vi "Calibration.vi"(0 "Mode":T3, 5 "Calib file":path, 9 "Simulate/Run":T2) -> (14 "Calib const":string[][](array[string]), 16 "Coefficients":dbl[][](array[numeric]) format="%.2f", 19 "Status Out":T1)   [LabVIEW 2015]
uses:
  Anemometry Sub Vis/Globals/Calib_global.vi
  Anemometry Sub Vis/Globals/Meas_global.vi
  Anemometry Sub Vis/Controls/Setup.ctl
  Anemometry Sub Vis/Controls/Post_Process.ctl
  Anemometry Sub Vis/Gen Trav/Multi_Run_Status.ctl
  Anemometry Sub Vis/Controls/App_Global.ctl
  Anemometry Sub Vis/Calibration/Calib_mode.ctl
  Anemometry Sub Vis/Controls/Save_Data.ctl
  Anemometry Sub Vis/Acquisition/PWA/PWAtasksGLOBAL.vi
  Anemometry Sub Vis/File/Setup_Filetype.ctl
  <vilib>/Analysis/NI_AALBase.lvlib
  <vilib>/Analysis/baseanly.llb/Mean (DBL).vi
  Anemometry Sub Vis/Controls/User_Specific_mode.ctl
panel:
  in  "-ve Ref Values":bool
  out "String":string
  in  "polynomial order":i32=2 min=1 max=3 step=1
  out "Ref velocity":dbl[](array[numeric])=[2.4275346736, 2.4395664609, 2.453235235, 2.4247395837, 2.4277603784, 2.41169823, 2.4254144559, 2.424896502176921] format="%.3f"
  out "labels":string[](array[string])=["XW1 Volt", "XW2 Volt", "Entered Val", "Selector"]
  in  "Point selector 3":cluster{"Y":dbl, "X":dbl, "t/f":bool}[](array[cluster]) {"X" format="%#.2g"; "Y" format="%#.3f"}
  in  "n":dbl=0.45 format="%.4f"
  in  "Fixed n":bool=TRUE
  out "Sample of input signals":dbl[][](graph)
  in  "Sampling speeds":T4={"Samples/ch"=600, "Sample Rate/ch (Hz)"=100.0} {"Sample Rate/ch (Hz)" min=0; "Samples/ch" min=0 step=1}
  out "Calibration plot":cluster{cluster{dbl, dbl}[]}[](graph)
  in  "Point selector 4":T5(array[cluster]) {"Y2" format="%#.2f"; "X" format="%#.3f"; "Y" format="%#.2f"}
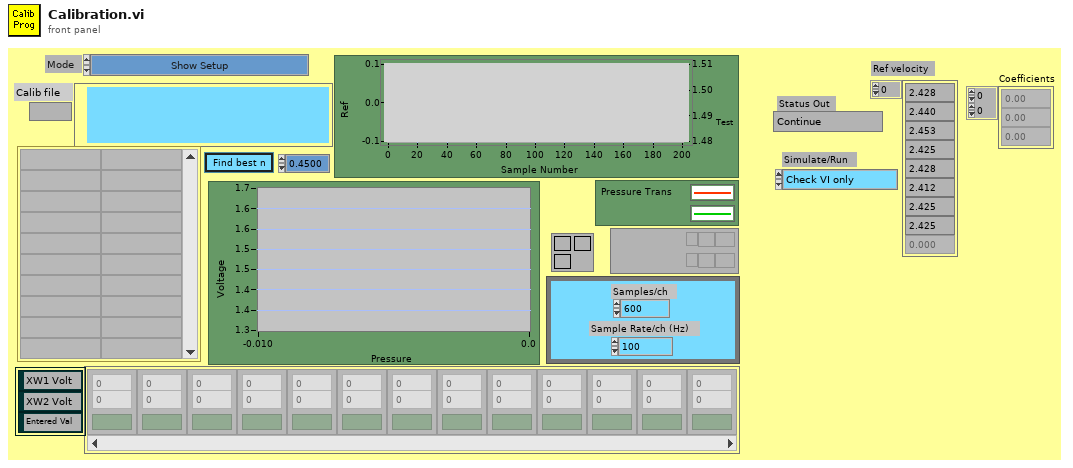
[diagram p1: front panel]
types:
  T1 = typedef "Multi_Run_Status.ctl" = enum16{"Continue", "Jump to Next Point", "Jump to Next Row", "Jump To Fall Back", "Terminate Run"}
  T2 = typedef "User_Specific_mode.ctl" = enum16{"Check VI only", "Run VI"}
  T3 = typedef "Calib_mode.ctl" = enum16{"Show Setup", "Take a New Calibration Point", "Refit Curve", "Setup Front Panel"}
  T4 = cluster{"Samples/ch":i32, "Sample Rate/ch (Hz)":sgl}
  T5 = cluster{"Y":dbl, "Y2":dbl, "X":dbl, "t/f":bool}[]
  T6 = typedef "Post_Process.ctl" = enum16{"Take New Data", "Post Process Raw Data File"}
  T7 = typedef "Setup_Filetype.ctl" = enum16{"Measurement Setups", "Calibration Setups", "General", "Results File Plotter Setups", "Speed Calib Tweaks"}
  T8 = typedef "Save_Data.ctl" = enum16{"Save No Data", "Save Data"}
  T9 = typedef "Setup.ctl" = enum16{"Run Program", "Show Setup", "Save Current Setup", "Setup Front Panel"}
  T10 = typedef "App_Global.ctl" = enum16{"Read Global", "Write to Global", "Initialise Array"}
  T11 = enum32{"existing file", "new file", "new or existing file", "existing dir", "new dir", "new or existing dir", "existing file (use LLBs)", "new file (use LLBs)", "new or existing file (use LLBs)", "new or existing file or directory (use LLBs)"}
  T12 = cluster{"Samples /ch":i32, "Sampling Rate /ch (Hz)":sgl}
  T13 = typedef "Cal_Inst_type.ctl" = enum16{"Propeller anemometer", "Pressure Transducer", "Hot wire", "Cross wire velocity", "Cross wire angle", "Generic Linear", "Generic Polynomial", "Generic BackPoly", "Fast FID", "Thermocouple", "Cold wire", "Pulsed Wire"}
  T14 = typedef "Ref_Inst_type.ctl" = enum16{"Propellor anemometer", "Pressure Transducer", "Raw voltage", "Pitot-static tube", "Preston tube", "Generic Linear", "Generic Polynomial", "Thermocouple", "LDA", "Enter Value", "ADAM Channel"}
  T15 = cluster{"2nd Ref type":T14, "2nd inst present":bool}
  T16 = typedef "Analysis_info_cluster.ctl" = cluster{"Colour":u32, "Inst type":T17, "Inst name":string, "Symbol":string, "Code name":string, "Extra Info":string, "Inst Array":T18, "Extra Titles":string[], "Extra Values":string[], "U":dbl, "u^2":dbl, "u^3":dbl, "u^4":dbl, "Skew_u":dbl, "Kurt_u":dbl, "Sd Error in Mean":dbl, "% u'/U":dbl, "X":dbl, "Y":dbl, "Z":dbl, "Timescale integral to 25%":dbl, "Sd Error in Variance":dbl, "Calib File":path, "Calib Constants":dbl[], "Output Position":bool, "Full Stats":bool, "Av Sampling Rate":dbl, "Av No of Samples":dbl, "Total Meas Time (s)":dbl, "ADAM Ch Name":string}
  T17 = typedef "Inst_type.ctl" = enum16{"Propeller anemometer", "Raw voltage", "Pressure Transducer", "Pitot-static tube", "Preston tube", "Hot wire", "Cross wire 1", "Cross wire 2", "Generic Linear", "Generic Polynomial", "Generic BackPoly", "Fast FID", "Thermocouple", "Cold wire", "Pulsed Wire", "LDA Vel", "LDA Tran time", "LDA Arr time", "Microphone"}
  T18 = typedef "Instrument_Array.ctl" = enum16{"PWA", "LDA", "Analogue"}
  T19 = typedef "Time_Trace_Cluster.ctl" = cluster{"Weighting":dbl[], "Time (s)":dbl[], "Voltage":dbl[], "Eng Values":dbl[]}
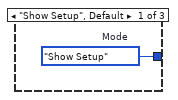
[diagram p5: hidden frame]
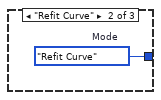
[diagram p6: hidden frame]
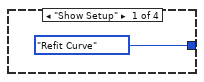
[diagram p7: hidden frame]
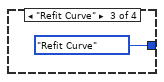
[diagram p8: hidden frame]
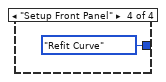
[diagram p9: hidden frame]
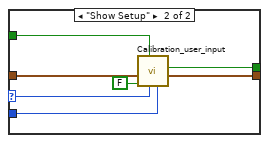
[diagram p14: hidden frame]
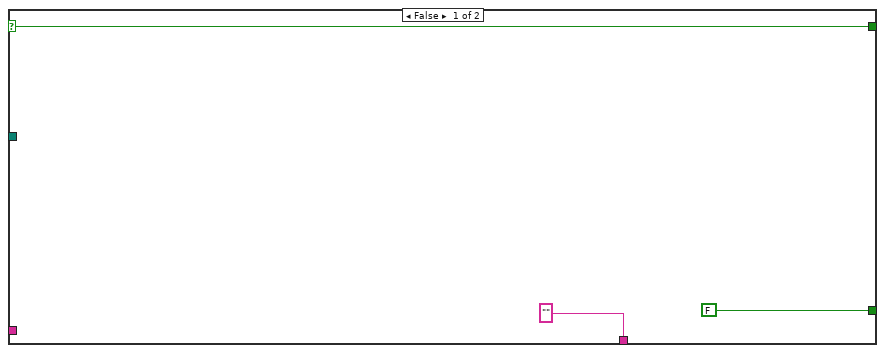
[diagram p15: hidden frame]
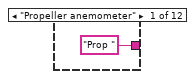
[diagram p16: hidden frame]
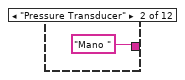
[diagram p17: hidden frame]
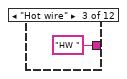
[diagram p18: hidden frame]
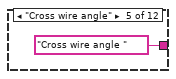
[diagram p19: hidden frame]
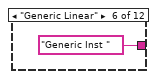
[diagram p20: hidden frame]
diagram:
  # "Change of file"
  # "Take new point"
  # "Calib File already valid"
  # "Main Calib File"
  # "Temp"
  # "Temp"
  # "Setup"
  # "E inst 1"
  # "Ref"
  # "E Inst 1\n+ 1 pt"
  # "Vel\n+1 pt"
  # "E inst 2"
  # "E Inst 2\n+ 1 pt"
  # "2nd ref"
  # "2nd ref"
  n1 = flat-sequence {
    tunnel: "Simulate/Run" -> [w106]
    tunnel: [w115] -> w101
    tunnel: [w120] -> w100
    tunnel: [w114] -> w99
    tunnel: w101 -> [w134]
    tunnel: [w134] -> w98
    tunnel: w100 -> [w129]
    tunnel: [w129] -> w97
    tunnel: [w136] -> w96
    tunnel: [w130] -> w95
    tunnel: [w133] -> w94
    tunnel: w99 -> [w128]
    tunnel: [w128] -> w93
    tunnel: w98 -> [w153]
    tunnel: [w153] -> w92
    tunnel: w97 -> [w152]
    tunnel: [w152] -> w91
    tunnel: w96 -> [w157]
    tunnel: [w157] -> w90
    tunnel: w95 -> [w156]
    tunnel: [w156] -> w89
    tunnel: w94 -> [w154]
    tunnel: [w154] -> w88
    tunnel: w93 -> [w151]
    tunnel: [w151] -> w87
    tunnel: [w189] -> w86
    tunnel: [w190] -> w85
    tunnel: w92 -> [w188]
    tunnel: [w188] -> w84
    tunnel: w91 -> [w187]
    tunnel: [w182] -> w83
    tunnel: w90 -> [w185]
    tunnel: [w185] -> w82
    tunnel: w89 -> [w184]
    tunnel: [w184] -> w81
    tunnel: w88 -> [w183]
    tunnel: [w183] -> w80
    tunnel: w87 -> [w186]
    tunnel: [w186] -> w79
    tunnel: w86 -> [w240]
    tunnel: [w240] -> w78
    tunnel: w85 -> [w239]
    tunnel: [w239] -> w77
    tunnel: w84 -> [w238]
    tunnel: [w238] -> w76
    tunnel: w83 -> [w237]
    tunnel: [w237] -> w75
    tunnel: w82 -> [w236]
    tunnel: [w236] -> w74
    tunnel: w81 -> [w235]
    tunnel: [w235] -> w73
    tunnel: w80 -> [w234]
    tunnel: [w234] -> w72
    tunnel: w79 -> [w233]
    tunnel: [w233] -> w71
    tunnel: w78 -> [w371]
    tunnel: [w371] -> w70
    tunnel: w77 -> [w370]
    tunnel: [w370] -> w69
    tunnel: w76 -> [w369]
    tunnel: [w369] -> w68
    tunnel: w75 -> [w368]
    tunnel: [w368] -> w67
    tunnel: w74 -> [w367]
    tunnel: [w367] -> w66
    tunnel: w73 -> [w366]
    tunnel: [w366] -> w65
    tunnel: w72 -> [w365]
    tunnel: [w365] -> w64
    tunnel: w71 -> [w364]
    tunnel: [w364] -> w63
    tunnel: [w510] -> w62
    tunnel: [w509] -> w61
    tunnel: [w508] -> w60
    tunnel: [w507] -> w59
    tunnel: w70 -> [w496]
    tunnel: w69 -> [w497]
    tunnel: [w506] -> w58
    tunnel: w68 -> [w490]
    tunnel: [w490] -> w57
    tunnel: w67 -> [w489]
    tunnel: [w489] -> w56
    tunnel: w66 -> [w488]
    tunnel: [w488] -> w55
    tunnel: w65 -> [w487]
    tunnel: [w487] -> w54
    tunnel: [w498] -> w53
    tunnel: w64 -> [w486]
    tunnel: [w486] -> w52
    tunnel: w63 -> [w491]
    tunnel: w62 -> [w543]
    tunnel: [w543] -> w51
    tunnel: w61 -> [w542]
    tunnel: [w542] -> w50
    tunnel: w60 -> [w541]
    tunnel: [w541] -> w49
    tunnel: w59 -> [w540]
    tunnel: [w540] -> w48
    tunnel: w58 -> [w539]
    tunnel: [w539] -> w47
    tunnel: w57 -> [w538]
    tunnel: [w538] -> w46
    tunnel: w56 -> [w547]
    tunnel: w55 -> [w537]
    tunnel: [w537] -> w45
    tunnel: w54 -> [w536]
    tunnel: [w536] -> w44
    tunnel: w53 -> [w545]
    tunnel: w52 -> [w544]
    tunnel: w51 -> [w569]
    tunnel: [w569] -> w43
    tunnel: w50 -> [w568]
    tunnel: [w568] -> w42
    tunnel: w49 -> [w567]
    tunnel: [w567] -> w41
    tunnel: w48 -> [w566]
    tunnel: [w566] -> w40
    tunnel: w47 -> [w565]
    tunnel: [w565] -> w39
    tunnel: w46 -> [w564]
    tunnel: [w564] -> w38
    tunnel: w45 -> [w563]
    tunnel: [w563] -> w37
    tunnel: w44 -> [w571]
    tunnel: [w571] -> w36
    tunnel: w43 -> [w616]
    tunnel: [w616] -> w35
    tunnel: w42 -> [w615]
    tunnel: [w615] -> w34
    tunnel: w41 -> [w614]
    tunnel: [w614] -> w33
    tunnel: w40 -> [w613]
    tunnel: [w613] -> w32
    tunnel: [w620] -> w31
    tunnel: w39 -> [w612]
    tunnel: [w612] -> w30
    tunnel: w38 -> [w621]
    tunnel: [w621] -> w29
    tunnel: w37 -> [w611]
    tunnel: [w611] -> w28
    tunnel: w36 -> [w610]
    tunnel: [w610] -> w27
    tunnel: [w647] -> w26
    tunnel: [w646] -> w25
    tunnel: w35 -> [w649]
    tunnel: w34 -> [w648]
    tunnel: w33 -> [w644]
    tunnel: [w645] -> w24
    tunnel: w32 -> [w643]
    tunnel: [w642] -> w23
    tunnel: w31 -> [w635]
    tunnel: [w635] -> w22
    tunnel: [w640] -> w21
    tunnel: w30 -> [w633]
    tunnel: w29 -> [w638]
    tunnel: [w638] -> w20
    tunnel: w28 -> [w637]
    tunnel: [w637] -> w19
    tunnel: w27 -> [w634]
    tunnel: [w634] -> w18
    tunnel: w26 -> [w995]
    tunnel: w25 -> [w998]
    tunnel: [w998] -> w17
    tunnel: w24 -> [w997]
    tunnel: w23 -> [w992]
    tunnel: w22 -> [w990]
    tunnel: [w990] -> w16
    tunnel: w21 -> [w996]
    tunnel: w20 -> [w989]
    tunnel: [w989] -> w15
    tunnel: w19 -> [w988]
    tunnel: [w988] -> w14
    tunnel: w18 -> [w987]
    tunnel: [w987] -> w13
    tunnel: [w993] -> w12
    tunnel: [w991] -> w11
    tunnel: w17 -> [w1009]
    tunnel: [w1009] -> w10
    tunnel: w16 -> [w1008]
    tunnel: [w1008] -> w9
    tunnel: w15 -> [w1026]
    tunnel: [w1026] -> w8
    tunnel: w14 -> [w1007]
    tunnel: [w1007] -> w7
    tunnel: w13 -> [w1006]
    tunnel: [w1006] -> w6
    tunnel: w12 -> [w1010]
    tunnel: w11 -> [w1025]
    tunnel: w10 -> [w1042]
    tunnel: [w1042] -> w5
    tunnel: w9 -> [w1047]
    tunnel: w8 -> [w1039]
    tunnel: [w1039] -> w4
    tunnel: w7 -> [w1041]
    tunnel: [w1041] -> w3
    tunnel: w6 -> [w1040]
    tunnel: [w1040] -> w2
    tunnel: w5 -> [w1069]
    tunnel: w4 -> [w1070]
    tunnel: w3 -> [w1071]
    tunnel: w2 -> [w1068]
    tunnel: [w1068] -> w1
    tunnel: w1 -> [w1117]
    frame #0 {
      w104 = FALSE  # Visible
      # "Calib-Frame0-InitialSetup"
      n2 = case shown="\"Run VI\"" w106 {
        frame "Check VI only" {
        }
        frame "Run VI" {
          n3 = Current VI's Path() -> (path=w108:path)
          n4 = call "Open_Close_Front_Panel.ph.vi"("Front Panel Window:Open"=TRUE, "VI path"=w108) -> ()  [unwired: 2 out]
        }
      }
      n5 = call "Run_EnFlo_Hub.vi"() -> ()  [unwired: 8 out]
      n6 = property on="String" class="Str"("Visible"=w104, "Blinking"=w104) -> ()  [unwired: 2 in, 2 out]
      n7 = global write "Calib_global.vi" "New Setup String"("") -> ()
      n8 = global write "Meas_global.vi" "Raw data option"(enum16{"Save raw data", "Raw data not saved"}."Save raw data" ("Raw data option")) -> ()
      n9 = global write "Meas_global.vi" "Post Process"(Post_Process."Take New Data" ("Post Process")) -> ()
    }
    frame #1 {
      w121 = FALSE  # Warn if Already Exists
      # "Calib-Frame1-FrameDescription"
      n10 = call "Current_Filepath.vi"("Short_Name"="Cal" ("Data Type"), "Filename in"="Calib file", "Data Type"="Calibrations") -> ("Filename Out"=w112:path)  [unwired: 1 in, 1 out]
      n11 = Empty String/Path?(string/path=w112) -> (empty?=w117:bool)
      n12 = case shown="True" w117 {
        tunnel: w112 -> [w123 _]
        tunnel: [w123 w125] -> w119
        frame False {
        }
        frame True {
          (unwired) T11."new or existing file" ("select mode (2)")
          # "Why is this here?"
          n13 = File Dialog(7:"Please Choose a new or existing Calibration filename" ("Promp if not found")) -> (1:w124:bool, 3:w125:path)  [unwired: 1 in, 7 out]
          n14 = Stop(stop? (T)=w124) -> ()
        }
      }
      n15 = call "Results_filename_checker.vi"("Warn if Already Exists"=w121, "Comment"="for the Calibration Prog", "Results file"=w119) -> ("exists?"=w120:bool, "cancelled"=w118:bool, "Results file output"=w115:path)  [unwired: 2 in, 1 out]
      n16 = Stop(stop? (T)=w118) -> ()
      n17 = global write "Calib_global.vi" "Calib file"(w115) -> ()
      n18 = local write "Calib file"(w115) -> ()
      n19 = global write "Meas_global.vi" "Results file"(w115) -> ()
      n20 = Format Into String(format string="Calibration File   %s", w115) -> (resulting string=w114:string)  [unwired: 2 in, 1 out]
    }
    frame #2 {
      # "Calib-Frame2-FrameDescription"
      n21 = while {
        shift-right: [w145] -> _
        shift-left: _ -> [w146]
        tunnel: w134 -> [w145]
        tunnel: [w144] -> w133
        stop <- FALSE continue-if-true
        n22 = Not Equal?(x=w146, y=w145) -> (x != y?=w144:bool)
      }
      n23 = Current VI's Path() -> (path=w135:path)
      n24 = call "Running_as_top_level.vi"("Vi path name"=w135) -> ("Top Level"=w127:bool)  [unwired: 1 out]
      n25 = Compound Arithmetic op=AND(w133, w127) -> (w132:bool)
      n26 = case shown="True" w132 {
        tunnel: "Mode" -> [w137 w138]
        tunnel: [w137 w139] -> w130
        frame False {
        }
        frame True {
          n27 = case shown="\"Setup Front Panel\"" w138 {
            selector: w138 -> [_ _ w142]
            tunnel: [w140 w141 w142] -> w139
            frame "Show Setup", Default {
              w140 = Calib_mode."Show Setup"  # Mode
            }
            frame "Refit Curve" {
              w141 = Calib_mode."Refit Curve"  # Mode
            }
            frame "Setup Front Panel" {
            }
          }
        }
      }
      n28 = case shown="\"Take a New Calibration Point\"" w130 {
        tunnel: [enum16{"Take new data point", "Refit Curve"}."Refit Curve" ("data mode") enum16{"Take new data point", "Refit Curve"}."Take new data point" ("data mode") enum16{"Take new data point", "Refit Curve"}."Refit Curve" ("data mode") enum16{"Take new data point", "Refit Curve"}."Refit Curve" ("data mode")] -> w136
        frame "Show Setup" {
        }
        frame "Take a New Calibration Point" {
        }
        frame "Refit Curve" {
        }
        frame "Setup Front Panel" {
        }
      }
    }
    frame #3 {
      # "The code in these two cases is essentially duplicated. Only,\nthe input to the Boolean input named \"OK\" differs between\nthe two cases. We should be able either flatten this out, or\nuse the case structure to only alter the input to the \"OK\"\ninput of Calibration_user_input.vi."
      # "Calib-Frame3-FrameDescription"
      n29 = local read "Fixed n"() -> (w159:bool)
      n30 = case shown="\"Setup Front Panel\"" w156 {
        tunnel: [w162 w163 TRUE w165] -> w155
        tunnel: w154 -> [w162 w163 _ w165]
        frame "Show Setup" {
        }
        frame "Refit Curve" {
        }
        frame "Setup Front Panel" {
        }
        frame "Take a New Calibration Point" {
        }
      }
      n31 = case shown="\"Take a New Calibration Point\", Default" w156 {
        selector: w156 -> [w168 w175]
        tunnel: "Sampling speeds" -> [w174 w181]
        tunnel: w157 -> [w172 w179]
        tunnel: [w171 w178] -> w160
        tunnel: w159 -> [w169 w177]
        tunnel: [w170 w176] -> w158
        frame "Take a New Calibration Point", Default {
          n32 = call "Calibration_user_input.vi"("data mode"=w172, "Mode"=w168, "Fixed n"=w169, "OK"=TRUE, "Sampling speeds"=w174) -> ("Sampling speeds Output"=w171:T12, "Fixed n out"=w170:bool)  [unwired: 2 in, 3 out]
        }
        frame "Show Setup" {
          n33 = call "Calibration_user_input.vi"("data mode"=w179, "Mode"=w175, "Fixed n"=w177, "OK"=FALSE, "Sampling speeds"=w181) -> ("Sampling speeds Output"=w178:T12, "Fixed n out"=w176:bool)  [unwired: 5 out]
        }
      }
      n34 = case shown="True" w155 {
        tunnel: w160 -> [_ w167]
        tunnel: w158 -> [_ w166]
        frame False {
        }
        frame True {
          n35 = local write "Sampling speeds"(w167) -> ()
          n36 = local write "Fixed n"(w166) -> ()
        }
      }
    }
    frame #4 {
      # "Calib-Frame4-FrameDescription"
      n37 = case shown="True" w187 {
        selector: w187 -> [w191 w194]
        tunnel: ["" ("Output string") w209] -> w190
        tunnel: [FALSE w208] -> w189
        tunnel: w188 -> [_ w200]
        tunnel: w186 -> [_ w195]
        tunnel: [w191 w194] -> w182
        frame False {
        }
        frame True {
          w199 = FALSE  # Show Dialog?
          n38 = global read "Calib_global.vi" "Instrument type"() -> (w203:T13)
          n39 = case shown="\"Cross wire velocity\"" w203 {
            tunnel: ["Prop " "Mano " "HW " "Cross wire velocity " "Cross wire angle " "Generic Inst " "Generic Polynomial " "Generic BackPoly " "Fast FID " "Thermocouple " "Cold wire " "Pulsed wire "] -> w204
            frame "Propeller anemometer" {
            }
            frame "Pressure Transducer" {
            }
            frame "Hot wire" {
            }
            frame "Cross wire velocity" {
            }
            frame "Cross wire angle" {
            }
            frame "Generic Linear" {
            }
            frame "Generic Polynomial" {
            }
            frame "Generic BackPoly" {
            }
            frame "Fast FID" {
            }
            frame "Thermocouple" {
            }
            frame "Cold wire" {
            }
            frame "Pulsed Wire" {
            }
          }
          n40 = call "Read_Characters_From_File.ph.vi"("file path (dialog if empty)"=w200, "number of characters (all:-1)"=-1) -> ("character string"=w197:string)  [unwired: 7 out]
          n41 = Concatenate Strings(w204, "calib label") -> (w205:string)
          n42 = Concatenate Strings("\r", w197) -> (w196:string)
          n43 = call "Get_string_subset.vi"("String Name"=w195, "Show Dialog?"=w199, "String to split"=w196, "File Label"=w205) -> ("Status"=w202:enum16{"Char in string", "Char not in string"}, "Output string"=w201:string)
          n44 = case shown="\"Char in string\"" w202 {
            tunnel: w201 -> [w228 _]
            tunnel: [w228 ""] -> w209
            tunnel: [w223 FALSE] -> w208
            tunnel: w195 -> [w222 _]
            frame "Char in string" {
              w229 = FALSE  # Show Dialog?
              n45 = call "2D_array_from_string.vi"("String Name"=w222, "Show Dialog?"=w229, "Input string"=w228, "Array title"="Calib points label") -> ("2D data array"=w227:dbl[][])
              n46 = Array Size(array=w227) -> (size(s)=w226:i32[])
              n47 = Index Array(array=w226, index=0 ("Index")) -> (element=w224:i32)
              n48 = Greater Than 0?(x=w224) -> (x > 0?=w223:bool)
            }
            frame "Char not in string" {
            }
          }
        }
      }
    }
    frame #5 {
      w243 = ""
      # "Calib-Frame5-FrameDescription"
      n49 = global read "Calib_global.vi" "Ref Instrument type"() -> (w251:T14)
      n50 = global read "Calib_global.vi" "2nd ref instrument"() -> (w250:T15)
      n51 = global read "Calib_global.vi" "Instrument type"() -> (w254:T13)
      n52 = case shown="\"Propellor anemometer\"" w251 {
        tunnel: [w280 w283 w287 w289 w292 w295 w298 w301 w304 string[] [] string[] []] -> w247
        tunnel: [FALSE FALSE FALSE FALSE TRUE FALSE FALSE FALSE FALSE FALSE FALSE] -> w242
        frame "Propellor anemometer" {
          n53 = Build Array("Prop Velocity") -> (w280:string[])
        }
        frame "Pressure Transducer" {
          n54 = Build Array("Pressure Trans") -> (w283:string[])
        }
        frame "Raw voltage" {
          n55 = Build Array("Raw Voltage") -> (w287:string[])
        }
        frame "Pitot-static tube" {
          n56 = Build Array("Pitot Vel") -> (w289:string[])
        }
        frame "Preston tube" {
          n57 = Build Array("Shear stress") -> (w292:string[])
        }
        frame "Generic Linear" {
          n58 = Build Array("Gen Lin") -> (w295:string[])
        }
        frame "Generic Polynomial" {
          n59 = Build Array("Gen Poly") -> (w298:string[])
        }
        frame "Thermocouple" {
          n60 = Build Array("Thermo") -> (w301:string[])
        }
        frame "LDA" {
          n61 = Build Array("LDA Vel") -> (w304:string[])
        }
        frame "Enter Value" {
        }
        frame "ADAM Channel" {
        }
      }
      n62 = case shown="\"Propeller anemometer\"" w254 {
        tunnel: [w314 w318 w322 w326 w331 w336 w340 w344 w348 w352 w356 w361] -> w244
        tunnel: [FALSE FALSE FALSE FALSE FALSE FALSE TRUE TRUE FALSE FALSE TRUE TRUE] -> w246
        tunnel: [w312 w316 w320 w324 w329 w334 w338 w342 w346 w350 w354 FALSE] -> w241
        tunnel: w242 -> [w312 w316 w320 w324 w329 w334 w338 w342 w346 w350 w354 _]
        frame "Propeller anemometer" {
          n63 = Build Array("Prop Voltage") -> (w314:string[])
        }
        frame "Pressure Transducer" {
          n64 = Build Array("Pressure Trans") -> (w318:string[])
        }
        frame "Hot wire" {
          n65 = Build Array("HW Voltage") -> (w322:string[])
        }
        frame "Cross wire velocity" {
          n66 = Build Array("XW1 Voltage", "XW2 Voltage") -> (w326:string[])
        }
        frame "Cross wire angle" {
          n67 = Build Array("XW1 Voltage", "XW2 Voltage") -> (w331:string[])
        }
        frame "Generic Linear" {
          n68 = Build Array("Generic Voltage") -> (w336:string[])
        }
        frame "Generic Polynomial" {
          n69 = Build Array("Generic Voltage") -> (w340:string[])
        }
        frame "Generic BackPoly" {
          n70 = Build Array("Generic Voltage") -> (w344:string[])
        }
        frame "Fast FID" {
          n71 = Build Array("FF Voltage") -> (w348:string[])
        }
        frame "Thermocouple" {
          n72 = Build Array("Thermo Voltage") -> (w352:string[])
        }
        frame "Cold wire" {
          n73 = Build Array("CW Voltage") -> (w356:string[])
        }
        frame "Pulsed Wire" {
          n74 = local write "polynomial order"(3 ("polynomial order")) -> ()
          n75 = Build Array("PWA 1/TOF") -> (w361:string[])
        }
      }
      n76 = Unbundle By Name(w250) -> ("2nd Ref type"=w248:T14, "2nd inst present"=w249:bool)
      n77 = case shown="True" w249 {
        tunnel: w248 -> [_ w257]
        tunnel: [w256 w258] -> w245
        tunnel: w247 -> [w256 _]
        frame False {
        }
        frame True {
          n78 = case shown="\"Propellor anemometer\"" w257 {
            tunnel: [w259 w261 w264 w265 w267 w269 w271 w273 w275 string[] [] string[] []] -> w258
            frame "Propellor anemometer" {
              n79 = Build Array("Prop Velocity") -> (w259:string[])
            }
            frame "Pressure Transducer" {
              n80 = Build Array("Pressure Trans") -> (w261:string[])
            }
            frame "Raw voltage" {
              n81 = Build Array("Raw Voltage") -> (w264:string[])
            }
            frame "Pitot-static tube" {
              n82 = Build Array("Pitot Vel") -> (w265:string[])
            }
            frame "Preston tube" {
              n83 = Build Array("Shear stress") -> (w267:string[])
            }
            frame "Generic Linear" {
              n84 = Build Array("Gen Lin") -> (w269:string[])
            }
            frame "Generic Polynomial" {
              n85 = Build Array("Gen Poly") -> (w271:string[])
            }
            frame "Thermocouple" {
              n86 = Build Array("Thermo") -> (w273:string[])
            }
            frame "LDA" {
              n87 = Build Array("LDA Vel") -> (w275:string[])
            }
            frame "Enter Value" {
            }
            frame "ADAM Channel" {
            }
          }
        }
      }
      n88 = case shown="False" w241 {
        frame False {
          n89 = local write "-ve Ref Values"(FALSE ("-ve Ref Values")) -> ()
        }
        frame True {
        }
      }
      n90 = property on="-ve Ref Values" class="Bool (strict)"("Visible"=w241) -> ()  [unwired: 2 in, 2 out]
      n91 = property on="polynomial order" class="DigNum (strict)"("Visible"=w246) -> ()  [unwired: 2 in, 2 out]
      n92 = Build Array (concatenate)(w245, w244, w243, w243, w243) -> (w252:string[])
      n93 = for {
        N: 3 -> [_]
        tunnel: w252 -> [w310] mode=indexing
        i -> [w311]
        n94 = property on="Sample of input signals" class="WFGraph (strict)"("Active Plot"=w311, "Plot.Plot Name"=w310) -> ()  [unwired: 2 in, 2 out]
      }
    }
    frame #6 {
      # "Calib-Frame6-FrameDescription"
      n95 = global read "Calib_global.vi" "Ref Instrument type"() -> (w374:T14)
      n96 = case shown="\"Propellor anemometer\"" w374 {
        tunnel: ["Prop Vel" "Pressure" "Voltage" "Pitot Vel" "Shear stress" "Generic Linear" "Generic Poly" "Thermo T" "LDA Vel" "Entered Val" "ADAM Channel"] -> w377
        frame "Propellor anemometer" {
        }
        frame "Pressure Transducer" {
        }
        frame "Raw voltage" {
        }
        frame "Pitot-static tube" {
        }
        frame "Preston tube" {
        }
        frame "Generic Linear" {
        }
        frame "Generic Polynomial" {
        }
        frame "Thermocouple" {
        }
        frame "LDA" {
        }
        frame "Enter Value" {
        }
        frame "ADAM Channel" {
        }
      }
      n97 = global read "Calib_global.vi" "Instrument type"() -> (w375:T13)
      n98 = case shown="\"Propeller anemometer\"" w375 {
        tunnel: [FALSE FALSE TRUE TRUE TRUE FALSE FALSE FALSE FALSE FALSE FALSE FALSE] -> w363
        tunnel: [TRUE TRUE TRUE FALSE FALSE TRUE TRUE TRUE TRUE TRUE TRUE TRUE] -> w379
        tunnel: [FALSE FALSE FALSE TRUE TRUE FALSE FALSE FALSE FALSE FALSE FALSE FALSE] -> w378
        tunnel: w377 -> [w392 w399 w408 w418 w428 w438 w444 w451 w458 w466 w472 w479]
        tunnel: [w395 w402 w411 w421 w431 w440 w447 w454 w461 w468 w475 w482] -> w376
        tunnel: "Selector" -> [w394 w401 w410 w420 w430 w437 w446 w453 w460 w465 w474 w481]
        tunnel: [w393 w400 "E^2" "XW Volt^2" "Y" w439 w444 w452 w458 w467 w472 w479] -> w372
        tunnel: [w392 w399 w406 w416 "X" w438 w445 w451 w459 w466 w473 w480] -> w373
        frame "Propeller anemometer" {
          w393 = "Prop Volt"
          n99 = Build Array(w393, w392, w394) -> (w395:string[])
        }
        frame "Pressure Transducer" {
          w400 = "Voltage"
          n100 = Build Array(w400, w399, w401) -> (w402:string[])
        }
        frame "Hot wire" {
          n101 = Concatenate Strings(w408, "^n") -> (w406:string)
          n102 = Build Array("HW Volt", w408, w410) -> (w411:string[])
        }
        frame "Cross wire velocity" {
          n103 = Concatenate Strings(w418, "^n") -> (w416:string)
          n104 = Build Array("XW1 Volt", "XW2 Volt", w418, w420) -> (w421:string[])
        }
        frame "Cross wire angle" {
          n105 = Build Array("XW1 Volt", "XW2 Volt", w428, w430) -> (w431:string[])
        }
        frame "Generic Linear" {
          w439 = "Gen Volt"
          n106 = Build Array(w439, w438, w437) -> (w440:string[])
        }
        frame "Generic Polynomial" {
          w445 = "Gen Volt"
          n107 = Build Array(w445, w444, w446) -> (w447:string[])
        }
        frame "Generic BackPoly" {
          w452 = "Gen Volt"
          n108 = Build Array(w451, w452, w453) -> (w454:string[])
        }
        frame "Fast FID" {
          w459 = "FF Volt"
          n109 = Build Array(w459, w458, w460) -> (w461:string[])
        }
        frame "Thermocouple" {
          w467 = "Thermo Volt"
          n110 = Build Array(w467, w466, w465) -> (w468:string[])
        }
        frame "Cold wire" {
          w473 = "CW Volt"
          n111 = Build Array(w473, w472, w474) -> (w475:string[])
        }
        frame "Pulsed Wire" {
          w480 = "1/TOF"
          n112 = Build Array(w480, w479, w481) -> (w482:string[])
        }
      }
      "labels" <- w376
      n113 = property on="Calibration plot" class="XYGraph (strict)"("X Scale.Name Label.Text"=w373, "Y Scale.Name Label.Text"=w372) -> ()  [unwired: 2 in, 2 out]
      n114 = property on="Point selector 3" class="Arr (strict)"("Visible"=w379) -> ()  [unwired: 2 in, 2 out]
      n115 = property on="Point selector 4" class="Arr (strict)"("Visible"=w378) -> ()  [unwired: 2 in, 2 out]
      n116 = property on="Fixed n" class="Bool (strict)"("Visible"=w363) -> ()  [unwired: 2 in, 2 out]
      n117 = property on="n" class="DigNum (strict)"("Visible"=w363) -> ()  [unwired: 2 in, 2 out]
    }
    frame #7 {
      # "Case structure to read previous calibration points if required"
      # "Calib-Frame7-FrameDescription"
      n118 = global read "Calib_global.vi" "Calibration Points"() -> (w495:dbl[])
      n119 = case shown="True" w496 {
        tunnel: w497 -> [_ w530]
        tunnel: [w522 w527] -> w494
        tunnel: w495 -> [w523 w526]
        tunnel: w491 -> [_ w524]
        frame False {
          n120 = Build Array(w523) -> (w522:dbl[][])
        }
        frame True {
          w529 = FALSE  # Show Dialog?
          n121 = Array Size(array=w526) -> (size(s)=w525:i32)
          n122 = call "2D_array_from_string.vi"("String Name"=w524, "Show Dialog?"=w529, "Input string"=w530, "Array title"="Calib points label") -> ("2D data array"=w528:dbl[][])
          n123 = case shown="1, Default" w525 {
            tunnel: w528 -> [w532 w535]
            tunnel: [w532 w534] -> w527
            tunnel: w526 -> [_ w533]
            frame 0 {
            }
            frame 1, Default {
              n124 = Build Array (concatenate)(w535, w533) -> (w534:dbl[][])
            }
          }
        }
      }
      n125 = for {
        tunnel: w494 -> [w511] mode=indexing
        shift-right: [w512] -> w492
        shift-left: dbl[][] [] -> [w513]
        n126 = Array Subset(array=w511, length=2) -> (w516:dbl[])  [unwired: 1 in]
        n127 = Not A Number/Path/Refnum?(number/path/refnum=w516) -> (NaN/Path/Refnum?=w515:bool[])
        n128 = Or Array Elements(Boolean array=w515) -> (logical OR=w514:bool)
        n129 = case shown="False" w514 {
          tunnel: w513 -> [w520 w521]
          tunnel: w511 -> [w519 _]
          tunnel: [w518 w521] -> w512
          frame False {
            n130 = Build Array (concatenate)(w520, w519) -> (w518:dbl[][])
          }
          frame True {
          }
        }
      }
      n131 = Index Array(array=w492, index (col)=0) -> (element=w509:dbl[])  [unwired: 1 in]
      n132 = Index Array(array=w492, index (col)=1) -> (element=w510:dbl[])  [unwired: 1 in]
      n133 = Index Array(array=w492, index (col)=2) -> (element=w508:dbl[])  [unwired: 1 in]
      n134 = Index Array(array=w492, index (col)=3) -> (element=w507:dbl[])  [unwired: 1 in]
      n135 = Index Array(array=w492, index (col)=4) -> (element=w506:dbl[])  [unwired: 1 in]
      n136 = Index Array(array=w492, index (col)=5) -> (element=w499:dbl[])  [unwired: 1 in]
      n137 = Not A Number/Path/Refnum?(number/path/refnum=w499) -> (NaN/Path/Refnum?=w498:bool[])
    }
    frame #8 {
      # "Calib-Frame8-FrameDescription"
      n138 = And(x=w544, y=w547) -> (x .and. y?=w546:bool)
      n139 = case shown="True" w546 {
        tunnel: w545 -> [_ w548]
        frame False {
        }
        frame True {
          n140 = local read "Point selector 3"() -> (w552:cluster{"Y":dbl, "X":dbl, "t/f":bool}[])
          n141 = local read "Point selector 4"() -> (w549:T5)
          n142 = for {
            tunnel: w552 -> [w560]
            tunnel: [w562] -> w551 mode=indexing
            tunnel: w548 -> [w561] mode=indexing
            i -> [w559]
            n143 = Index Array(array=w560, index=w559) -> (element=w558:cluster{"Y":dbl, "X":dbl, "t/f":bool})
            n144 = Bundle By Name(cluster=w558, "t/f"=w561) -> (w562:cluster{"Y":dbl, "X":dbl, "t/f":bool})
          }
          n145 = for {
            tunnel: w549 -> [w555]
            tunnel: [w557] -> w550 mode=indexing
            tunnel: w548 -> [w556] mode=indexing
            i -> [w554]
            n146 = Index Array(array=w555, index=w554) -> (element=w553:cluster{"Y":dbl, "Y2":dbl, "X":dbl, "t/f":bool})
            n147 = Bundle By Name(cluster=w553, "t/f"=w556) -> (w557:cluster{"Y":dbl, "Y2":dbl, "X":dbl, "t/f":bool})
          }
          n148 = local write "Point selector 3"(w551) -> ()
          n149 = local write "Point selector 4"(w550) -> ()
        }
      }
    }
    frame #9 {
      w574 = "Setup for instrument being calibrated"
      # "Calib-Frame9-FrameDescription"
      n150 = global read "Calib_global.vi" "Pre Setup String"() -> (w572:string)
      n151 = case shown="\"Show Setup\"" w571 {
        tunnel: w572 -> [w579 w583]
        tunnel: w574 -> [w578 w582]
        tunnel: [w577 w581] -> w573
        tunnel: "Previous Setup String" ("String Name") -> [w576 w580]
        frame "Take a New Calibration Point", Default {
          n152 = call "Get_string_subset.vi"("String Name"=w576, "String to split"=w579, "File Label"=w578) -> ("Output string"=w577:string)  [unwired: 1 in, 1 out]
        }
        frame "Show Setup" {
          n153 = call "Get_string_subset.vi"("String Name"=w580, "String to split"=w583, "File Label"=w582) -> ("Status"=w585:enum16{"Char in string", "Char not in string"}, "Output string"=w586:string)  [unwired: 1 in]
          n154 = case shown="\"Char not in string\"" w585 {
            tunnel: [w588 w589] -> w584
            tunnel: w586 -> [w588 _]
            tunnel: w583 -> [_ w589]
            frame "Char in string" {
            }
            frame "Char not in string" {
            }
          }
          n155 = global read "Calib_global.vi" "Instrument type"() -> (w587:T13)
          n156 = case shown="\"Hot wire\"" w587 {
            tunnel: [w591 w593 w596 w599 w602 w604 w606 w608 ""] -> w581
            tunnel: w584 -> [w590 w592 w594 w597 w600 w603 w605 w607 _]
            frame "Propeller anemometer" {
              n157 = call "Propeller_setup.vi"("Setup String"=w590) -> ("Output string"=w591:string)
            }
            frame "Pressure Transducer" {
              n158 = call "Pressure_Transducer_Setup.vi"("Setup String"=w592) -> ("Output string"=w593:string)
            }
            frame "Hot wire" {
              n159 = call "Hot_Wire_Setup.vi"("XW?"=FALSE, "Setup String"=w594) -> ("Output string"=w596:string)
            }
            frame "Cross wire velocity" {
              n160 = call "Hot_Wire_Setup.vi"("XW?"=TRUE, "Setup String"=w597) -> ("Output string"=w599:string)
            }
            frame "Cross wire angle" {
              n161 = call "Hot_Wire_Setup.vi"("XW?"=TRUE, "Setup String"=w600) -> ("Output string"=w602:string)
            }
            frame "Generic Linear" {
              n162 = call "Generic_setup.vi"("Setup String"=w603) -> ("Output String"=w604:string)
            }
            frame "Generic Polynomial" {
              n163 = call "Generic_setup.vi"("Setup String"=w605) -> ("Output String"=w606:string)
            }
            frame "Generic BackPoly" {
              n164 = call "Generic_setup.vi"("Setup String"=w607) -> ("Output String"=w608:string)
            }
            frame "Fast FID", Default {
            }
          }
        }
      }
      n165 = call "Add_label_to_string.vi"("String to write"=w573, "File Label"=w574) -> ("Output string"=w575:string)
      n166 = global write "Calib_global.vi" "Instument setup Info"(w575) -> ()
    }
    frame #10 {
      w622 = TRUE  # Lock File
      w628 = FALSE  # advisory dialog? (display:T)
      w629 = FALSE  # append to file? (new file:F)
      # "Calib-Frame10-FrameDescription"
      n167 = Path To String(path=w621) -> (string=w623:string)
      n168 = call "Date_and_Time_to_string.vi"() -> ("Date and time (spreadsheet)"=w631:string)
      n169 = call "Characters_to_string.vi"("Characters to write"=w623, "Label for characters"="Calib filename") -> ("Output string"=w632:string)
      n170 = global read "Calib_global.vi" "Instument setup Info"() -> (w624:string)
      n171 = global read "Calib_global.vi" "New Setup String"() -> (w625:string)
      n172 = Concatenate Strings(w631, w632, w625, w624) -> (w620:string)
      n173 = call "Calib_read_files.vi"() -> ()  [unwired: 1 out]
      n174 = call "Setup_Filepath.vi"("Setup File Type"=Setup_Filetype."Calibration Setups", "Filename in"="Current_Setup.xls") -> ("Filename Out"=w617:path)  [unwired: 1 out]
      n175 = call "Add_label_to_string.vi"("String to write"=w620, "File Label"="Raw data header") -> ("Output string"=w626:string)
      n176 = call "Write_Characters_To_File.vi"("file path (dialog if empty)"=w617, "advisory dialog? (display:T)"=w628, "character string"=w626, "append to file? (new file:F)"=w629, "Lock File"=w622) -> ()  [unwired: 4 out]
    }
    frame #11 {
      # "Case structure for the decision 'MORE POINTS' or 'REFIT CURVE'"
      n177 = global read "Calib_global.vi" "2nd ref instrument"() -> (w641:T15)
      n178 = global read "Calib_global.vi" "Instrument type"() -> (w636:T13)
      n179 = case shown="\"Take new data point\"" w637 {
        tunnel: [w737 w986] -> w646
        tunnel: [w738 w982] -> w647
        tunnel: w649 -> [w739 w986]
        tunnel: w648 -> [w740 w982]
        tunnel: [w736 w985] -> w645
        tunnel: w644 -> [w735 w985]
        tunnel: w643 -> [w734 w984]
        tunnel: [w732 w984] -> w642
        tunnel: w641 -> [w733 _]
        tunnel: [w730 w983] -> w640
        tunnel: w633 -> [w731 w983]
        tunnel: w638 -> [w729 _]
        tunnel: [w728 Multi_Run_Status."Continue" ("Status Out")] -> w639
        tunnel: w636 -> [w727 _]
        frame "Take new data point" {
          # "Taking data for another calibration point"
          # "Start"
          n180 = flat-sequence {
            tunnel: w739 -> [w748]
            tunnel: [w748] -> w726
            tunnel: w740 -> [w747]
            tunnel: [w747] -> w725
            tunnel: w735 -> [w746]
            tunnel: [w746] -> w724
            tunnel: w734 -> [w745]
            tunnel: [w745] -> w723
            tunnel: w733 -> [w744]
            tunnel: [w744] -> w722
            tunnel: w731 -> [w743]
            tunnel: [w743] -> w721
            tunnel: w729 -> [w742]
            tunnel: [w742] -> w720
            tunnel: w727 -> [w741]
            tunnel: [w741] -> w719
            tunnel: [w752] -> w718
            tunnel: w726 -> [w759]
            tunnel: [w759] -> w717
            tunnel: w725 -> [w758]
            tunnel: [w758] -> w716
            tunnel: w724 -> [w757]
            tunnel: [w757] -> w715
            tunnel: w723 -> [w756]
            tunnel: [w756] -> w714
            tunnel: w722 -> [w755]
            tunnel: [w755] -> w713
            tunnel: w721 -> [w764]
            tunnel: [w763] -> w712
            tunnel: w720 -> [w761]
            tunnel: [w762] -> w711
            tunnel: w719 -> [w754]
            tunnel: [w754] -> w710
            tunnel: w718 -> [w753]
            tunnel: [w753] -> w709
            tunnel: w717 -> [w796]
            tunnel: [w796] -> w708
            tunnel: w716 -> [w795]
            tunnel: [w795] -> w707
            tunnel: w715 -> [w794]
            tunnel: [w794] -> w706
            tunnel: w714 -> [w793]
            tunnel: [w793] -> w705
            tunnel: w713 -> [w792]
            tunnel: [w792] -> w704
            tunnel: w712 -> [w791]
            tunnel: [w791] -> w703
            tunnel: w711 -> [w790]
            tunnel: [w790] -> w702
            tunnel: w710 -> [w789]
            tunnel: [w789] -> w701
            tunnel: w709 -> [w788]
            tunnel: [w788] -> w700
            tunnel: [w800] -> w699
            tunnel: [w798] -> w698
            tunnel: w708 -> [w821]
            tunnel: [w821] -> w697
            tunnel: w707 -> [w820]
            tunnel: [w820] -> w696
            tunnel: w706 -> [w819]
            tunnel: [w819] -> w695
            tunnel: w705 -> [w818]
            tunnel: [w818] -> w694
            tunnel: w704 -> [w817]
            tunnel: [w817] -> w693
            tunnel: w703 -> [w816]
            tunnel: [w816] -> w692
            tunnel: w702 -> [w815]
            tunnel: [w815] -> w691
            tunnel: w701 -> [w824]
            tunnel: [w824] -> w690
            tunnel: w700 -> [w814]
            tunnel: [w814] -> w689
            tunnel: w699 -> [w813]
            tunnel: [w813] -> w688
            tunnel: w698 -> [w812]
            tunnel: [w812] -> w687
            tunnel: [w825] -> w686
            tunnel: [w823] -> w685
            tunnel: [w822] -> w684
            tunnel: [w811] -> w683
            tunnel: w697 -> [w849]
            tunnel: [w849] -> w682
            tunnel: [w859] -> w681
            tunnel: w696 -> [w858]
            tunnel: w695 -> [w848]
            tunnel: [w848] -> w680
            tunnel: w694 -> [w847]
            tunnel: [w847] -> w679
            tunnel: w693 -> [w846]
            tunnel: [w846] -> w678
            tunnel: w692 -> [w845]
            tunnel: [w845] -> w677
            tunnel: w691 -> [w844]
            tunnel: [w844] -> w676
            tunnel: w690 -> [w843]
            tunnel: [w843] -> w675
            tunnel: [w856] -> w674
            tunnel: w689 -> [w857]
            tunnel: [w857] -> w673
            tunnel: w688 -> [w842]
            tunnel: [w842] -> w672
            tunnel: w687 -> [w841]
            tunnel: [w841] -> w671
            tunnel: w686 -> [w852]
            tunnel: w685 -> [w840]
            tunnel: [w840] -> w670
            tunnel: w684 -> [w839]
            tunnel: [w839] -> w669
            tunnel: w683 -> [w838]
            tunnel: [w838] -> w668
            tunnel: w682 -> [w871]
            tunnel: [w871] -> w667
            tunnel: w681 -> [w870]
            tunnel: [w870] -> w666
            tunnel: w680 -> [w869]
            tunnel: [w869] -> w665
            tunnel: w679 -> [w878]
            tunnel: [w877] -> w664
            tunnel: w678 -> [w876]
            tunnel: w677 -> [w868]
            tunnel: [w868] -> w663
            tunnel: w676 -> [w864]
            tunnel: [w864] -> w662
            tunnel: w675 -> [w873]
            tunnel: [w873] -> w661
            tunnel: w674 -> [w863]
            tunnel: w673 -> [w875]
            tunnel: w672 -> [w867]
            tunnel: [w867] -> w660
            tunnel: [w863] -> w659
            tunnel: w671 -> [w874]
            tunnel: [w874] -> w658
            tunnel: w670 -> [w866]
            tunnel: [w866] -> w657
            tunnel: w669 -> [w865]
            tunnel: [w865] -> w656
            tunnel: w668 -> [w872]
            tunnel: w667 -> [w917]
            tunnel: w666 -> [w907]
            tunnel: [w907] -> w655
            tunnel: [w916] -> w654
            tunnel: [w915] -> w653
            tunnel: w665 -> [w914]
            tunnel: w664 -> [w906]
            tunnel: [w906] -> w652
            tunnel: w663 -> [w905]
            tunnel: [w905] -> w651
            tunnel: w662 -> [w904]
            tunnel: [w904] -> w650
            tunnel: w661 -> [w910]
            tunnel: w660 -> [w913]
            tunnel: w659 -> [w912]
            tunnel: w658 -> [w911]
            tunnel: w657 -> [w909]
            tunnel: w656 -> [w908]
            tunnel: [w977] -> w738
            tunnel: w655 -> [w977]
            tunnel: [w976] -> w737
            tunnel: w654 -> [w976]
            tunnel: [w975] -> w736
            tunnel: w653 -> [w975]
            tunnel: [w974] -> w732
            tunnel: w652 -> [w974]
            tunnel: [w973] -> w730
            tunnel: w651 -> [w973]
            tunnel: [w972] -> w728
            tunnel: w650 -> [w972]
            frame #0 {
              w749 = TRUE  # Visible
              w750 = "Currently Taking a New Calibration Point"  # String
              n181 = Get Date/Time In Seconds() -> (seconds since 1Jan1904=w751:timestamp)
              n182 = property on="String" class="Str"("Visible"=w749, "Blinking"=w749) -> ()  [unwired: 2 in, 2 out]
              n183 = To Double Precision Float(number=w751) -> (double precision float=w752:dbl)
              "String" <- w750
            }
            frame #1 {
              # "Acquire data from input channels"
              n184 = while {
                tunnel: [w770] -> w762
                tunnel: w761 -> [w769]
                stop <- w768 continue-if-true
                n185 = flat-sequence {
                  tunnel: w769 -> [w771]
                  tunnel: [w771] -> w767
                  tunnel: [w774] -> w766
                  tunnel: w767 -> [w778]
                  tunnel: [w774] -> w765
                  tunnel: [w782] -> w770
                  tunnel: w766 -> [w782]
                  tunnel: [w784] -> w768
                  tunnel: w765 -> [w783]
                  frame #0 {
                    n186 = global write "Meas_global.vi" "Remote control"(TRUE ("Remote control")) -> ()
                  }
                  frame #1 {
                    n187 = call "Get_Data_Base_file_code.vi"("Data Type"="Raw_Calibrations", "Results Filename"=w778, "Short_Name"="Raw_Cal" ("Data Type")) -> ("Raw Data File Name"=w775:path)  [unwired: 1 in, 3 out]
                    n188 = call "Measurement.vi"("setup"=Setup."Run Program", "Post Process"=Post_Process."Take New Data", "File"=Save_Data."Save No Data", "Raw data file"=w775, "Setup filename"="Calib_Setup.xls") -> ("Status Out"=w774:T1)  [unwired: 2 in, 12 out]
                  }
                  frame #2 {
                    n189 = global read "Meas_global.vi" "Repeat Measurement?"() -> (w785:bool)
                    n190 = Equal?(x=w783, y=Multi_Run_Status."Continue" ("Status Out")) -> (x = y?=w786:bool)
                    n191 = And(x=w786, y=w785) -> (x .and. y?=w784:bool)
                  }
                }
              }
              n192 = global read "Calib_global.vi" "Temp (deg C)"() -> (w760:dbl)
              n193 = Build Array (concatenate)(w764, w760) -> (w763:dbl[])
            }
            frame #2 {
              n194 = global read "Meas_global.vi" "Analysis Info cluster"() -> (w800:T16[])
              n195 = global read "Meas_global.vi" "Time Trace"() -> (w797:T19[])
              n196 = for {
                tunnel: w800 -> [w806] mode=indexing
                shift-right: [w803] -> w798
                shift-left: dbl[][] [] -> [w804]
                tunnel: w797 -> [w802] mode=indexing
                n197 = Unbundle By Name(w806) -> ("Inst Array"=w805:T18)
                n198 = Unbundle By Name(w802) -> ("Eng Values"=w801:dbl[])
                n199 = case shown="\"Analogue\"" w805 {
                  tunnel: w804 -> [w807 w810]
                  tunnel: w801 -> [_ w809]
                  tunnel: [w807 w808] -> w803
                  frame "PWA", Default {
                  }
                  frame "Analogue" {
                    n200 = Build Array (concatenate)(w810, w809) -> (w808:dbl[][])
                  }
                }
              }
              "Sample of input signals" <- w798
            }
            frame #3 {
              n201 = case shown="\"Pulsed Wire\"" w824 {
                tunnel: [0 ("Index in") 1 ("Index in")] -> w825
                tunnel: [w826 w829] -> w823
                tunnel: [w826 w833] -> w822
                tunnel: [w826 w832] -> w811
                frame "Propeller anemometer", Default {
                  w826 = 0.0 ("mean")
                }
                frame "Pulsed Wire" {
                  n202 = global read "PWAtasksGLOBAL.vi" "PWA 1/TOF"() -> (w836:dbl[][])
                  n203 = Index Array(array=w836, index (row)=0) -> (element=w834:dbl[])  [unwired: 1 in]
                  n204 = call "Mean_fr_NaN_data.vi"("Data"=w834) -> ("Mean value"=w829:dbl)  [unwired: 1 out]
                  n205 = Multiply(x=w834, y=w834) -> (x*y=w831:dbl[])
                  n206 = Less Than 0?(x=w829) -> (x < 0?=w828:bool)
                  n207 = call "Mean_fr_NaN_data.vi"("Data"=w831) -> ("Mean value"=w833:dbl)  [unwired: 1 out]
                  n208 = Multiply(x=w834, y=w831) -> (x*y=w830:dbl[])
                  n209 = local write "-ve Ref Values"(w828) -> ()
                  n210 = call "Mean_fr_NaN_data.vi"("Data"=w830) -> ("Mean value"=w832:dbl)  [unwired: 1 out]
                }
              }
            }
            frame #4 {
              # "Adding the velocity\nvalue to the array"
              n211 = global read "Calib_global.vi" "ADAM Channel Name"() -> (w850:string)
              n212 = global read "Calib_global.vi" "Ref Instrument type"() -> (w855:T14)
              n213 = call "Get_ref_inst_value.vi"("Ref Instrument type"=w855, "ADAM Channel Name"=w850, "Index in"=w852, "Start time"=w857) -> ("Ref Value"=w854:dbl, "Index out"=w856:i32)  [unwired: 3 in, 7 out]
              n214 = case shown="True" "-ve Ref Values" {
                tunnel: w854 -> [w860 w862]
                tunnel: [w860 w861] -> w853
                frame False {
                }
                frame True {
                  n215 = Negate(x=w862) -> (-x=w861:dbl)
                }
              }
              n216 = Build Array (concatenate)(w858, w853) -> (w859:dbl[])
            }
            frame #5 {
              n217 = Unbundle(w876) -> ("2nd Ref type"=w880:T14, "2nd inst present"=w879:bool)
              n218 = case shown="True" w879 {
                tunnel: w863 -> [w886 w900]
                tunnel: [w884 w901] -> w881
                tunnel: w880 -> [_ w902]
                tunnel: w875 -> [_ w903]
                tunnel: w874 -> [w885 _]
                tunnel: w873 -> [w883 _]
                tunnel: w872 -> [w882 _]
                frame False {
                  n219 = case shown="\"Fast FID\"" w883 {
                    tunnel: w886 -> [_ _ w897 _]
                    tunnel: w885 -> [_ _ w896 _]
                    tunnel: [0.0 ("mean") w888 w894 w898] -> w884
                    tunnel: w882 -> [_ _ _ w898]
                    frame "Propeller anemometer", Default {
                    }
                    frame "Fast FID" {
                      n220 = Build Array("GMU:Source:ppm/%Density") -> (w891:string[])
                      n221 = call "Get_Channel_averages.vi"("Desired Ch Names"=w891, "Averaging time (mins)"=0.2) -> ("number"=w889:dbl[])  [unwired: 1 in, 2 out]
                      n222 = Index Array(array=w889) -> (element=w888:dbl)  [unwired: 1 in]
                    }
                    frame "Generic Polynomial" {
                      n223 = Index Array(array=w896, index (row)=w897) -> (element=w893:dbl[])  [unwired: 1 in]
                      n224 = Compound Arithmetic op=MULTIPLY(w893, w893, w893) -> (w895:dbl[])
                      n225 = call-poly <vilib>:"Mean.vi"("X"=w895) -> ("mean"=w894:dbl)  [unwired: 1 out]
                    }
                    frame "Pulsed Wire" {
                    }
                  }
                }
                frame True {
                  n226 = global read "Calib_global.vi" "ADAM Channel Name Vel Ref"() -> (w899:string)
                  n227 = call "Get_ref_inst_value.vi"("Ref Instrument type"=w902, "ADAM Channel Name"=w899, "Index in"=w900, "Start time"=w903) -> ("Ref Value"=w901:dbl)  [unwired: 4 in, 7 out]
                }
              }
              n228 = Build Array (concatenate)(w878, w881) -> (w877:dbl[])
            }
            frame #6 {
              n229 = case shown="\"Cross wire velocity\"" w910 {
                tunnel: w917 -> [w922 w932 w939 w947 w959 w970]
                tunnel: [w923 w933 w940 w948 w960 w971] -> w916
                tunnel: w914 -> [w921 w931 w938 w943 w958 w969]
                tunnel: [w921 w930 w937 w941 w957 w968] -> w915
                tunnel: w913 -> [w919 _ _ w945 w953 w964]
                tunnel: w912 -> [w924 w934 _ w949 w951 w962]
                tunnel: w911 -> [_ w929 _ _ _ _]
                tunnel: w909 -> [_ _ w936 _ _ _]
                tunnel: w908 -> [_ _ w935 _ _ _]
                frame "Propeller anemometer", Default {
                  n230 = Index Array(array=w919, index=w924) -> (element=w920:T16)
                  n231 = Unbundle By Name(w920) -> ("U"=w918:dbl)
                  n232 = Build Array (concatenate)(w922, w918) -> (w923:dbl[])
                }
                frame "Generic Polynomial" {
                  n233 = Index Array(array=w929, index (row)=w934) -> (element=w926:dbl[])  [unwired: 1 in]
                  n234 = Multiply(x=w926, y=w926) -> (x*y=w925:dbl[])
                  n235 = call-poly <vilib>:"Mean.vi"("X"=w926) -> ("mean"=w928:dbl)  [unwired: 1 out]
                  n236 = call-poly <vilib>:"Mean.vi"("X"=w925) -> ("mean"=w927:dbl)  [unwired: 1 out]
                  n237 = Build Array (concatenate)(w932, w928) -> (w933:dbl[])
                  n238 = Build Array (concatenate)(w931, w927) -> (w930:dbl[])
                }
                frame "Pulsed Wire" {
                  n239 = Build Array (concatenate)(w939, w936) -> (w940:dbl[])
                  n240 = Build Array (concatenate)(w938, w935) -> (w937:dbl[])
                }
                frame "Fast FID" {
                  n241 = Index Array(array=w945, index=w949) -> (element=w946:T16)
                  n242 = Unbundle By Name(w946) -> ("U"=w944:dbl, "u^2"=w942:dbl)
                  n243 = Build Array (concatenate)(w947, w944) -> (w948:dbl[])
                  n244 = Build Array (concatenate)(w943, w942) -> (w941:dbl[])
                }
                frame "Cross wire velocity" {
                  n245 = Increment(x=w951) -> (x+1=w950:i32)
                  n246 = Index Array(array=w953, index=w951) -> (element=w956:T16)
                  n247 = Index Array(array=w953, index=w950) -> (element=w955:T16)
                  n248 = Unbundle By Name(w956) -> ("U"=w952:dbl)
                  n249 = Unbundle By Name(w955) -> ("U"=w954:dbl)
                  n250 = Build Array (concatenate)(w959, w952) -> (w960:dbl[])
                  n251 = Build Array (concatenate)(w958, w954) -> (w957:dbl[])
                }
                frame "Cross wire angle" {
                  n252 = Increment(x=w962) -> (x+1=w961:i32)
                  n253 = Index Array(array=w964, index=w962) -> (element=w967:T16)
                  n254 = Index Array(array=w964, index=w961) -> (element=w966:T16)
                  n255 = Unbundle By Name(w967) -> ("U"=w963:dbl)
                  n256 = Unbundle By Name(w966) -> ("U"=w965:dbl)
                  n257 = Build Array (concatenate)(w970, w963) -> (w971:dbl[])
                  n258 = Build Array (concatenate)(w969, w965) -> (w968:dbl[])
                }
              }
            }
            frame #7 {
              w978 = FALSE  # Visible
              n259 = global read "Meas_global.vi" "Raw data file"() -> (w980:path)
              n260 = Strip Path(path=w980) -> (stripped path=w979:path)  [unwired: 1 out]
              n261 = property on="String" class="Str"("Visible"=w978, "Blinking"=w978) -> ()  [unwired: 2 in, 2 out]
              n262 = global write "Calib_global.vi" "Calib Raw Data Folder"(w979) -> ()
            }
          }
        }
        frame "Refit Curve" {
          # "Another calibration point is not\nrequired. Also  checks if there are\nany points to fit curve to."
        }
      }
      "Status Out" <- w639
    }
    frame #12 {
      # "Calib-Frame12-FrameDescription"
      n263 = Build Array(w995, w998, w997, w992, w996) -> (w994:dbl[][])
      n264 = call "Sort_Array_Indicies.vi"("unsorted array"=w995) -> ("Sort Index"=w991:i32[])  [unwired: 1 out]
      n265 = for {
        tunnel: w991 -> [w1001]
        tunnel: w994 -> [w1000] mode=indexing
        tunnel: [w999] -> w993 mode=indexing
        n266 = for {
          tunnel: w1001 -> [w1004] mode=indexing
          tunnel: w1000 -> [w1003]
          tunnel: [w1002] -> w999 mode=indexing
          n267 = Index Array(array=w1003, index=w1004) -> (element=w1002:dbl)
        }
      }
      "Ref velocity" <- w992
    }
    frame #13 {
      w1017 = FALSE  # t/f
      w1018 = FALSE  # t/f
      # "Calib-Frame13-FrameDescription"
      n268 = Index Array(array="Point selector 3", index=0) -> (element=w1023:cluster{"Y":dbl, "X":dbl, "t/f":bool})
      n269 = Index Array(array="Point selector 4", index=0) -> (element=w1015:cluster{"Y":dbl, "Y2":dbl, "X":dbl, "t/f":bool})
      n270 = Bundle By Name(cluster=w1023, "t/f"=w1018) -> (w1019:cluster{"Y":dbl, "X":dbl, "t/f":bool})
      n271 = Bundle By Name(cluster=w1015, "t/f"=w1017) -> (w1016:cluster{"Y":dbl, "Y2":dbl, "X":dbl, "t/f":bool})
      n272 = Build Array (concatenate)("Point selector 4", w1016) -> (w1012:T5)
      n273 = Build Array (concatenate)("Point selector 3", w1019) -> (w1021:cluster{"Y":dbl, "X":dbl, "t/f":bool}[])
      n274 = for {
        tunnel: w1021 -> [w1038]
        tunnel: w1025 -> [w1035] mode=indexing
        tunnel: [w1037] -> w1022 mode=indexing
        tunnel: w1012 -> [w1036]
        tunnel: [w1034] -> w1011 mode=indexing
        n275 = Index Array(array=w1038, index=w1035) -> (element=w1037:cluster{"Y":dbl, "X":dbl, "t/f":bool})
        n276 = Index Array(array=w1036, index=w1035) -> (element=w1034:cluster{"Y":dbl, "Y2":dbl, "X":dbl, "t/f":bool})
      }
      n277 = call "Calib_Analyse_fit.vi"("Calib file"=w1026, "Input points"=w1010, "polynomial order"="polynomial order", "Fixed n"="Fixed n", "n"="n", "Point selector 3"=w1022, "Point selector 4"=w1011) -> ("Calib const"=→"Calib const":string[][], "Calibration plot"=→"Calibration plot":cluster{cluster{dbl, dbl}[]}[], "Point selector 3 out"=w1031:cluster{"Y":dbl, "X":dbl, "t/f":bool}[], "Coefficients"=→"Coefficients":dbl[][], "Point selector 4 out"=w1030:T5)  [unwired: 4 out]
      n278 = local write "Point selector 3"(w1031) -> ()
      n279 = local write "Point selector 4"(w1030) -> ()
    }
    frame #14 {
      w1057 = FALSE  # Lock File
      w1059 = FALSE  # advisory dialog? (display:T)
      w1060 = FALSE  # append to file? (new file:F)
      # "Calib-Frame14-FrameDescription"
      n280 = global read "Calib_global.vi" "Calib Raw Data Folder"() -> (w1050:path)
      n281 = global read "Calib_global.vi" "Calib Raw Data Folder"() -> (w1051:path)
      n282 = Path To String(path=w1050) -> (string=w1049:string)
      n283 = call "Characters_to_string.vi"("Characters to write"=w1049, "Label for characters"="Calib Raw Data Folder") -> ("Output string"=w1046:string)
      n284 = global read "Calib_global.vi" "Header string"() -> (w1058:string)
      n285 = Concatenate Strings(w1047, w1046) -> (w1045:string)
      n286 = List Folder(path=w1051) -> (filenames=w1054:string[])  [unwired: 1 in, 5 out]
      n287 = Strip Path(path=w1039) -> (name=w1055:string)  [unwired: 1 out]
      n288 = call "Add_label_to_string.vi"("String to write"=w1045, "File Label"="Raw data header") -> ("Output string"=w1043:string)
      n289 = Array Size(array=w1054) -> (size(s)=w1053:i32)
      n290 = Concatenate Strings(w1058, w1043) -> (w1056:string)
      n291 = Greater Than 0?(x=w1053) -> (x > 0?=w1052:bool)
      n292 = case shown="True" w1052 {
        tunnel: w1056 -> [_ w1064]
        tunnel: w1055 -> [_ w1063]
        tunnel: w1051 -> [_ w1061]
        frame False {
        }
        frame True {
          w1065 = FALSE  # Lock File
          w1066 = FALSE  # append to file? (new file:F)
          w1067 = FALSE  # advisory dialog? (display:T)
          n293 = Build Path(base path=w1061, name or relative path=w1063) -> (appended path=w1062:path)
          n294 = call "Write_Characters_To_File.vi"("file path (dialog if empty)"=w1062, "advisory dialog? (display:T)"=w1067, "character string"=w1064, "append to file? (new file:F)"=w1066, "Lock File"=w1065) -> ()  [unwired: 4 out]
        }
      }
      n295 = call "Write_Characters_To_File.vi"("file path (dialog if empty)"=w1039, "advisory dialog? (display:T)"=w1059, "character string"=w1056, "append to file? (new file:F)"=w1060, "Lock File"=w1057) -> ()  [unwired: 4 out]
    }
    frame #15 {
      # "Calib-Frame15-FrameDescription"
      n296 = case shown="\"Take new data point\"" w1071 {
        tunnel: w1070 -> [w1077 _]
        tunnel: w1069 -> [w1073 _]
        frame "Take new data point" {
          n297 = global read "Calib_global.vi" "Calib Ch No"() -> (w1076:i16)
          n298 = flat-sequence {
            tunnel: w1077 -> [w1079]
            tunnel: [w1079] -> w1075
            tunnel: w1076 -> [w1080]
            tunnel: [w1080] -> w1074
            tunnel: w1073 -> [w1078]
            tunnel: [w1078] -> w1072
            tunnel: w1075 -> [w1096]
            tunnel: w1074 -> [w1090]
            tunnel: w1072 -> [w1089]
            frame #0 {
              n299 = Current VI's Path() -> (path=w1085:path)
              n300 = call "Running_as_top_level.vi"("Vi path name"=w1085) -> ("Top Level"=w1084:bool)  [unwired: 1 out]
              n301 = case shown="True" w1084 {
                frame False {
                }
                frame True {
                  n302 = call "Measurement.vi"("setup"=Setup."Setup Front Panel", "Post Process"=Post_Process."Take New Data", "File"=Save_Data."Save No Data") -> ()  [unwired: 4 in, 13 out]
                }
              }
              n303 = Build Array(w1080) -> (w1082:i16[])
              n304 = Build Array(w1079) -> (w1083:path[])
              n305 = call "Current_Calib_Filenames.vi"("Calib Filename"=w1083, "Channel Numbers"=w1082, "Mode"=App_Global."Write to Global") -> ()  [unwired: 3 out]
            }
            frame #1 {
              n306 = global read "Calib_global.vi" "Instrument type"() -> (w1098:T13)
              n307 = case shown="\"Cross wire angle\"" w1098 {
                tunnel: w1090 -> [_ w1110 w1116]
                tunnel: [path "" ("appended path") w1106 w1111] -> w1097
                tunnel: [FALSE TRUE TRUE] -> w1093
                frame "Propeller anemometer", Default {
                }
                frame "Cross wire angle" {
                  n308 = Format Into String(format string="Ch%d_XW_Angle_Calib", w1110) -> (resulting string=w1105:string)  [unwired: 2 in, 1 out]
                  n309 = call "Setup_Filepath.vi"("Setup File Type"=Setup_Filetype."Calibration Setups", "Filename in"=w1105) -> ("Filename Out"=w1106:path)  [unwired: 1 out]
                }
                frame "Cross wire velocity" {
                  n310 = Format Into String(format string="Ch%d_XW_Velocity_Calib", w1116) -> (resulting string=w1112:string)  [unwired: 2 in, 1 out]
                  n311 = call "Setup_Filepath.vi"("Setup File Type"=Setup_Filetype."Calibration Setups", "Filename in"=w1112) -> ("Filename Out"=w1111:path)  [unwired: 1 out]
                }
              }
              n312 = Array Size(array=w1089) -> (size(s)=w1095:i32)
              n313 = Greater?(x=w1095, y=1) -> (0:w1092:bool)
              n314 = And(x=w1092, y=w1093) -> (x .and. y?=w1091:bool)
              n315 = case shown="True" w1091 {
                tunnel: w1097 -> [_ w1101]
                tunnel: w1096 -> [_ w1100]
                frame False {
                }
                frame True {
                  n316 = call "Copy_with_Check.vi"("Mode"=enum16{"Move", "Copy"}."Copy", "Target Path"=w1101, "Variable Target?"=FALSE, "Source Path"=w1100) -> ()  [unwired: 1 out]
                }
              }
            }
          }
        }
        frame "Refit Curve" {
        }
      }
    }
    frame #16 {
      # "Calib-Frame16-FrameDescription"
      n317 = case shown="\"Show Setup\"" w1117 {
        frame "Show Setup" {
          n318 = local write "Mode"(Calib_mode."Take a New Calibration Point" ("Mode")) -> ()
        }
        frame "Take a New Calibration Point" {
        }
        frame "Refit Curve" {
        }
        frame "Setup Front Panel" {
          n319 = local write "Mode"(Calib_mode."Show Setup" ("Mode")) -> ()
        }
      }
      n320 = global write "Calib_global.vi" "Calibration Points"(dbl[] [] ("Calibration Points")) -> ()
    }
  }
